vi "Get All Local Control Refs.vi"(2 "Type":enum16{"Both", "Controls", "Indicators"}(ring)) -> (5 "VI Refnum":refnum<vi>, 6 "All Controls":refnum<vi>[](array[refnum]), 7 "Control Labels":string[](array[string]), 8 "error out":errorcluster)   [LabVIEW 2019]
doc: "This software is licensed for use under the “MIT License\"\nCopyright (c) 2019 Scott Hannahs, sth@alum.mit.edu\n\nPermission is hereby granted, free of charge, to any person obtaining a copy of this software and associated documentation files (the \"Software\"), to deal in the Software without restriction, including without limitation the rights to use, copy, modify, merge, publish, distribute, sublicense, and/or sell copies of the Software, and to permit persons to whom the Software is furnished to do so, subject to the following conditions: The above copyright notice and this permission notice shall be included in all copies or substantial portions of the Software.\n\nTHE SOFTWARE IS PROVIDED \"AS IS\", WITHOUT WARRANTY OF ANY KIND, EXPRESS OR IMPLIED, INCLUDING BUT NOT LIMITED TO THE WARRANTIES OF MERCHANTABILITY, FITNESS FOR A PARTICULAR PURPOSE AND NONINFRINGEMENT. IN NO EVENT SHALL THE AUTHORS OR COPYRIGHT HOLDERS BE LIABLE FOR ANY CLAIM, DAMAGES OR OTHER LIABILITY, WHETHER IN AN ACTION OF CONTRACT, TORT OR OTHERWISE, ARISING FROM, OUT OF OR IN CONNECTION WITH THE SOFTWARE OR THE USE OR OTHER DEALINGS IN THE SOFTWARE."
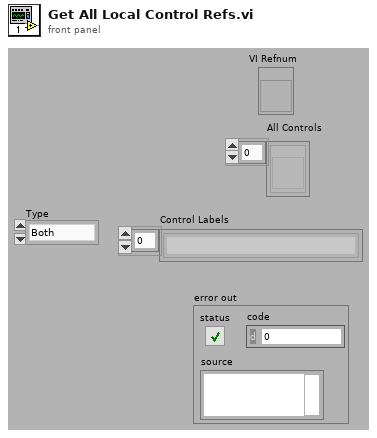
[diagram p1: front panel]
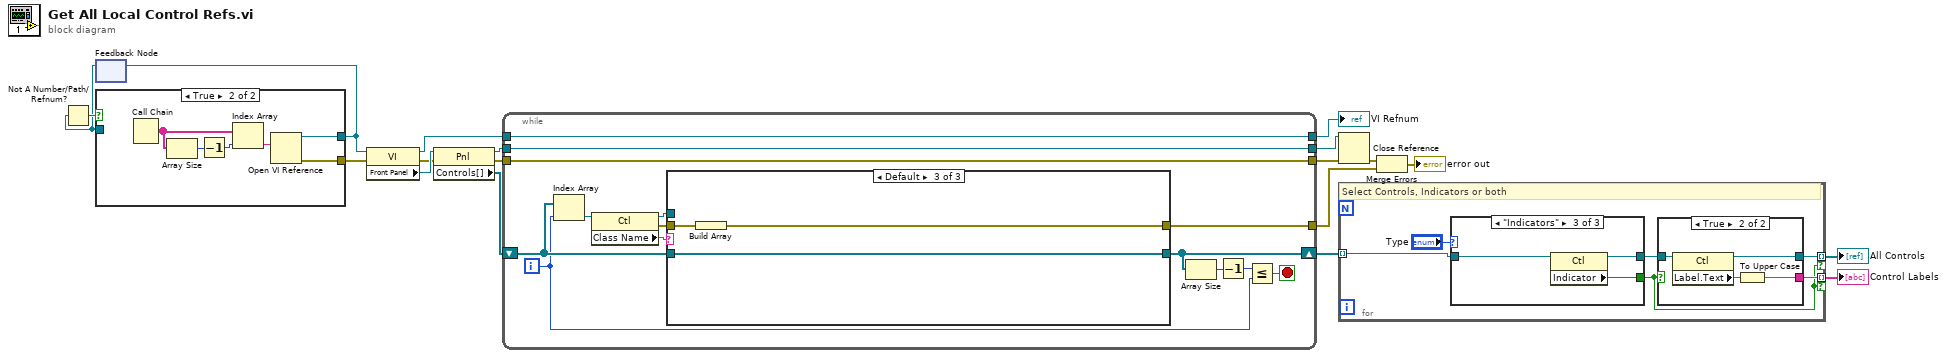
[diagram p0: block diagram]
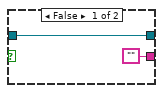
[diagram p2: hidden frame]
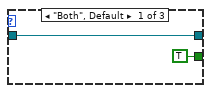
[diagram p3: hidden frame]
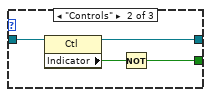
[diagram p4: hidden frame]
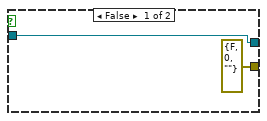
[diagram p5: hidden frame]
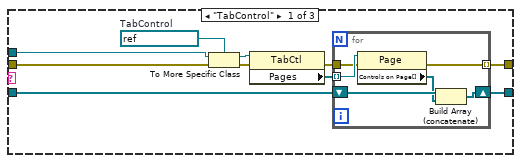
[diagram p6: hidden frame]
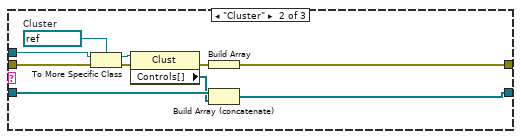
[diagram p7: hidden frame]
diagram:
  n1 = feedback #1() -> (w2:refnum<vi>)  [unwired: 1 in]
  n2 = Not A Number/Path/Refnum?(number/path/refnum=w2) -> (NaN/Path/Refnum?=w6:bool)
  n3 = case shown="True" w6 {
    tunnel: [w21 w27] -> w3
    tunnel: [errorcluster {"status"=FALSE, "code"=0, "source"=""} ("error out") w26] -> w18
    tunnel: w2 -> [w21 _]
    frame False {
    }
    frame True {
      n4 = Call Chain() -> (call chain=w25:string[])
      n5 = Array Size(array=w25) -> (size(s)=w24:i32)
      n6 = Decrement(x=w24) -> (x-1=w22:i32)
      n7 = Index Array(array=w25, index=w22) -> (element=w23:string)
      n8 = Open VI Reference(vi path=w23) -> (vi reference=w27:refnum<vi>, error out=w26:errorcluster)  [unwired: 5 in]
    }
  }
  n9 = feedback-in #1(w3) -> ()
  n10 = property class="VI"(reference=w3, error in=w18) -> (reference out=w8:refnum<vi>, error out=w13:errorcluster, "Front Panel"=w19:refnum<vi>)
  n11 = property class="Pnl"(reference=w19, error in=w13) -> (reference out=w11:refnum<vi>, error out=w9:errorcluster, "Controls[]"=w17:refnum<vi>[])
  n12 = while {
    shift-right: [w40] -> w4
    shift-left: w17 -> [w41]
    tunnel: [w31] -> w15
    tunnel: [w30] -> w12
    tunnel: w11 -> [w30]
    tunnel: w9 -> [w29]
    tunnel: [w29] -> w10
    tunnel: w8 -> [w28]
    tunnel: [w28] -> w7
    i -> [w38]
    stop <- w37 stop-if-true
    n13 = Index Array(array=w41, index=w38) -> (element=w35:refnum<vi>)
    n14 = property class="Ctl"(reference=w35) -> (reference out=w33:refnum<vi>, error out=w32:errorcluster, "Class Name"=w34:string)  [unwired: 1 in]
    n15 = case shown="Default" w34 {
      tunnel: w41 -> [w50 w67 w70]
      tunnel: [w49 w66 w70] -> w40
      tunnel: w33 -> [w48 w65 _]
      tunnel: w32 -> [w47 w64 w69]
      tunnel: [w42 w58 w68] -> w31
      frame "TabControl" {
        w44 = refnum<vi> refnum  # TabControl
        n16 = To More Specific Class(target class=w44, reference=w48, error in=w47) -> (specific class reference=w45:refnum<vi>, error out=w46:errorcluster)
        n17 = property class="TabCtl"(reference=w45, error in=w46) -> (error out=w43:errorcluster, "Pages"=w51:refnum<vi>[])  [unwired: 1 out]
        n18 = for {
          tunnel: w51 -> [w57] mode=indexing
          shift-right: [w56] -> w49
          shift-left: w50 -> [w55]
          tunnel: w43 -> [w53]
          tunnel: [w52] -> w42 mode=indexing
          n19 = property class="Page"(reference=w57, error in=w53) -> (error out=w52:errorcluster, "Controls on Page[]"=w54:refnum<vi>[])  [unwired: 1 out]
          n20 = Build Array (concatenate)(w55, w54) -> (w56:refnum<vi>[])
        }
      }
      frame "Cluster" {
        w61 = refnum<vi> refnum  # Cluster
        n21 = To More Specific Class(target class=w61, reference=w65, error in=w64) -> (specific class reference=w62:refnum<vi>, error out=w63:errorcluster)
        n22 = property class="Clust"(reference=w62, error in=w63) -> (error out=w59:errorcluster, "Controls[]"=w60:refnum<vi>[])  [unwired: 1 out]
        n23 = Build Array(w59) -> (w58:errorcluster[])
        n24 = Build Array (concatenate)(w67, w60) -> (w66:refnum<vi>[])
      }
      frame Default {
        n25 = Build Array(w69) -> (w68:errorcluster[])
      }
    }
    n26 = Array Size(array=w40) -> (size(s)=w39:i32)
    n27 = Decrement(x=w39) -> (x-1=w36:i32)
    n28 = Less Or Equal?(x=w36, y=w38) -> (x <= y?=w37:bool)
  }
  "VI Refnum" <- w7
  n29 = Close Reference(reference=w12, error in (no error)=w10) -> (error out=w14:errorcluster)
  n30 = for {
    tunnel: w4 -> [w76] mode=indexing
    tunnel: [w74] -> w5 mode=indexing if=w72
    tunnel: [w73] -> w1 mode=indexing if=w72
    # "Select Controls, Indicators or both"
    n31 = case shown="\"Indicators\"" "Type" {
      tunnel: w76 -> [w84 w88 w91]
      tunnel: [w84 w87 w89] -> w71
      tunnel: [TRUE ("Indicator") w85 w90] -> w72
      frame "Both", Default {
      }
      frame "Controls" {
        n32 = property class="Ctl"(reference=w88) -> (reference out=w87:refnum<vi>, "Indicator"=w86:bool)  [unwired: 1 in, 1 out]
        n33 = Not(x=w86) -> (.not. x?=w85:bool)
      }
      frame "Indicators" {
        n34 = property class="Ctl"(reference=w91) -> (reference out=w89:refnum<vi>, "Indicator"=w90:bool)  [unwired: 1 in, 1 out]
      }
    }
    n35 = case shown="True" w72 {
      tunnel: w71 -> [w78 w81]
      tunnel: [w78 w82] -> w74
      tunnel: ["" w79] -> w73
      frame False {
      }
      frame True {
        n36 = property class="Ctl"(reference=w81) -> (reference out=w82:refnum<vi>, "Label.Text"=w80:string)  [unwired: 1 in, 1 out]
        n37 = To Upper Case(1:w80) -> (0:w79:string)
      }
    }
  }
  "All Controls" <- w5
  "Control Labels" <- w1
  n38 = Merge Errors(w14, w15) -> (→"error out":errorcluster)
